vi "PH_TKTDS-30xx.PC Set Display Intensity.vi"(0 "i ref in":refnum<vi>, 2 "Intensity (1)":u8=1 min=1 max=100 step=1, 5 "error IO":errorcluster) -> (14 "i ref out":refnum<vi>, 19 "error out":errorcluster)   [LabVIEW 2014, in "PH_TKTDS-30xx.lvlib"]
doc: "This case sets the intensity of the waveforms at the display in percent."
uses:
  PH_TKTDS-30xx.lvlib
  instr.lib/TKDS3032-PHELIX/tktds3032-PHELIX - Driver np.lvlib
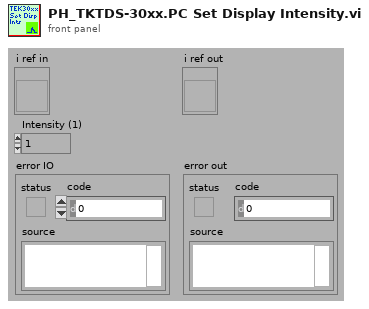
[diagram p1: front panel]
types:
  T1 = typedef "PH_TKTDS-30xx.lvlib/PH_TKTDS-30xx.i attribute.ctl" = cluster{"Default VISA Resource":string, "VISA Resource Name":refnum<visa-resource-name>, "Revision":cluster{"Instrument Driver":string, "Instrument Firmware":string}, "Selftest":cluster{"Result":u32, "Message":string}, "Channels":T2[], "Trigger Configuration":T3, "Acquisition Configuration":T4, "Fetched Waveforms":T5[], "GUI Refs":T6, "GUI Refs Channels":refnum<vi>[], "State":T7, "Error Message":string, "Allow Prdc Loop?":bool}
  T2 = typedef "PH_TKTDS-30xx.lvlib/PH_TKTDS-30xx.Channel Config.ctl" = cluster{"Channel Name":string, "Input Impedance":string, "Max Input Frequency":string, "Vertical Coupling":i32, "Channel Enabled":bool, "Probe Attenuation":dbl, "Vertical Range":dbl, "Vertical Offset":dbl}
  T3 = typedef "PH_TKTDS-30xx.lvlib/PH_TKTDS-30xx.Trigger Config.ctl" = cluster{"Source":string, "Slope":i32, "Level [V]":dbl}
  T4 = typedef "PH_TKTDS-30xx.lvlib/PH_TKTDS-30xx.Acquisition Config.ctl" = cluster{"Time base":dbl, "Record Length":u16, "Start Time":dbl, "Type":i32, "Continuous":bool}
  T5 = typedef "PH_TKTDS-30xx.lvlib/PH_TKTDS-30xx.fetched Waveform.ctl" = cluster{"Source":string, "Actual Points":u32, "Initial X":dbl, "X Increment":dbl, "Waveform Array":dbl[]}
  T6 = typedef "PH_TKTDS-30xx.lvlib/PH_TKTDS-30xx.GUI Refs.ctl" = cluster{"Trigger":refnum<vi>, "Acquisition":refnum<vi>, "Graph":refnum<vi>, "State":refnum<vi>, "Delete":refnum<vi>, "Channel to be positioned":refnum<vi>, "Postion":refnum<vi>, "Display Intensity":refnum<vi>, "VISA Resource":refnum<vi>}
  T7 = typedef "PH_StatusHandler.lvlib/PH_StatusHandler.Status.ctl" = i16
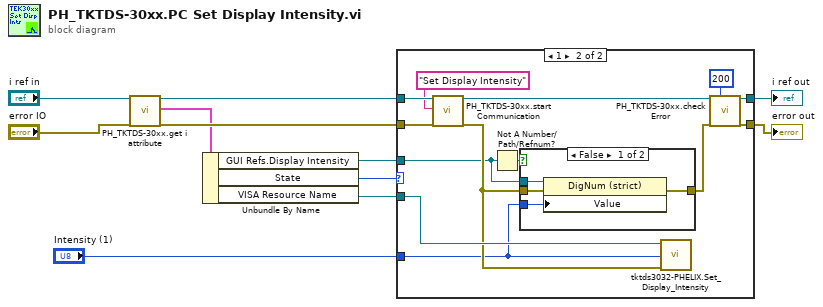
[diagram p0: block diagram]
diagram:
  n1 = call "PH_TKTDS-30xx.get i attribute.vi"("i ref in"="i ref in", "error in (no error)"="error IO") -> ("i ref out"=w6:refnum<vi>, "i attribute"=w8:T1, "error out"=w10:errorcluster)  [unwired: 15 in]
  n2 = Unbundle By Name(w8) -> ("GUI Refs.Display Intensity"=w3:refnum<vi>, "State"=w2:T7, "VISA Resource Name"=w9:refnum<visa-resource-name>)
  n3 = case shown="1" w2 {
    tunnel: w6 -> [w13 w26]
    tunnel: w9 -> [_ w25]
    tunnel: [w12 w24] -> w4
    tunnel: w10 -> [w12 w19]
    tunnel: [w13 w23] -> w11
    tunnel: w3 -> [_ w16]
    tunnel: "Intensity (1)" -> [_ w15]
    frame Default {
    }
    frame 1 {
      n4 = call "PH_TKTDS-30xx.start Communication.vi"("i ref in"=w26, "Action"="Set Display Intensity", "error in"=w19) -> ("i ref out"=w20:refnum<vi>, "error out"=w18:errorcluster)  [unwired: 15 in]
      n5 = Not A Number/Path/Refnum?(number/path/refnum=w16) -> (NaN/Path/Refnum?=w17:bool)
      n6 = case shown="False" w17 {
        tunnel: w18 -> [w30 w31]
        tunnel: [w29 w31] -> w14
        tunnel: w16 -> [w28 _]
        tunnel: w15 -> [w27 _]
        frame False {
          n7 = property class="DigNum (strict)"(reference=w28, error in=w30, "Value"=w27) -> (error out=w29:errorcluster)  [unwired: 1 out]
        }
        frame True {
        }
      }
      n8 = call "tktds3032-PHELIX.Set_Display_Intensity.vi"("error in (no error)"=w18, "Intensity (1)"=w15, "VISA Resource Name"=w25) -> ()  [unwired: 7 in, 2 out]
      n9 = call "PH_TKTDS-30xx.check Error.vi"("i ref in"=w20, "Waiting Time [ms]"=u32 200, "error in"=w14) -> ("i ref out"=w23:refnum<vi>, "error out"=w24:errorcluster)  [unwired: 15 in]
    }
  }
  "i ref out" <- w11
  "error out" <- w4
